vi "Rio_Testing_MoveXY (DONE).vi"() -> ()   [LabVIEW 2017]
panel:
  out "Counter Out 2":i32
  out "Counter Out":i32
  in  "Stop Button":bool
  in  "Boolean":bool
  out "Waveform Chart 2":dbl[][](graph)
  out "Waveform Chart":dbl[][](graph)
  out "Output Charts":T1
  in  "Home Position":dbl[](array[numeric])
  in  "Error In":errorcluster
  in  "Home/Coordinate (T/F)":bool
  in  "Coordinate":dbl[](array[numeric])
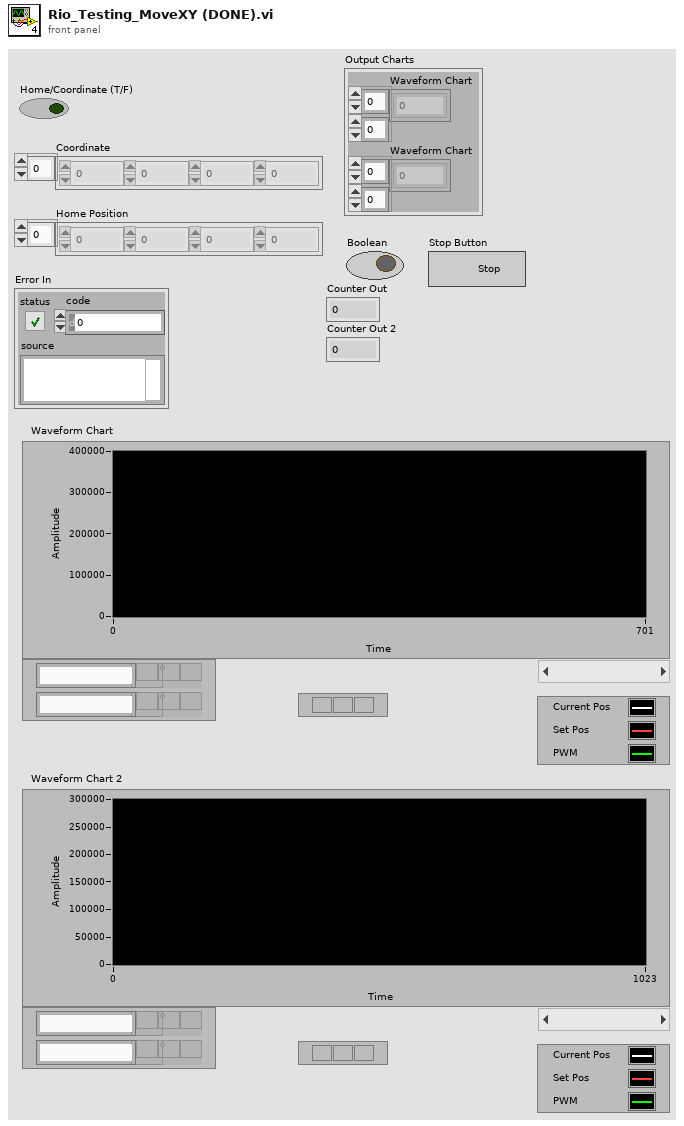
[diagram p1: front panel]
types:
  T1 = cluster{"Waveform Chart":dbl[][], "Waveform Chart":dbl[][]}
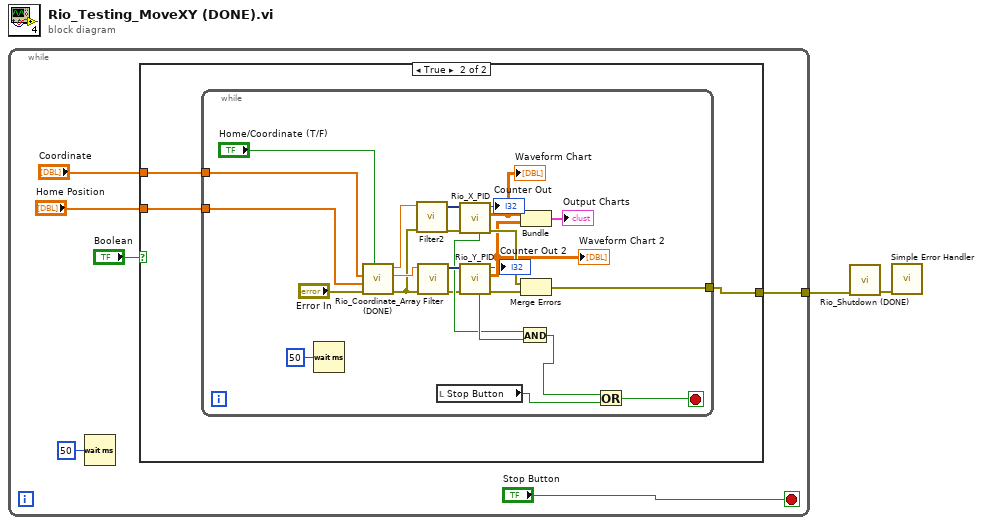
[diagram p0: block diagram]
diagram:
  n1 = while {
    tunnel: [w6] -> w1
    stop <- "Stop Button" stop-if-true
    n2 = Wait (ms)(milliseconds to wait=u32 50) -> ()  [unwired: 1 out]
    n3 = case shown="True" "Boolean" {
      tunnel: [_ w11] -> w6
      tunnel: "Home Position" -> [_ w10]
      tunnel: "Coordinate" -> [_ w9]
      frame False {
      }
      frame True {
        n4 = while {
          tunnel: [w22] -> w11
          tunnel: w10 -> [w19]
          tunnel: w9 -> [w18]
          stop <- w15 stop-if-true
          n5 = Wait (ms)(milliseconds to wait=u32 50) -> ()  [unwired: 1 out]
          n6 = call "Rio_Coordinate_Array (DONE).vi"("Coordinate Selection"="Home/Coordinate (T/F)", "Error In"="Error In", "Home Position"=w19, "Coordinate"=w18) -> ("Error Out"=w24:errorcluster, "Y"=w35:dbl, "X"=w23:dbl)  [unwired: 5 in]
          n7 = call "Filter2"("error in (no error)"=w24, "Signal"=w23) -> ("error out"=w25:errorcluster, "Filtered Signal"=w26:dynamicdata)  [unwired: 8 in]
          n8 = call "Filter"("error in (no error)"=w24, "Signal"=w35) -> ("error out"=w28:errorcluster, "Filtered Signal"=w33:dynamicdata)  [unwired: 8 in]
          n9 = local read "Stop Button"() -> (w14:bool)
          n10 = call "Rio_X_PID.vi"("Error In"=w25, "Setpoint"=w26) -> ("Error Out"=w29:errorcluster, "Waveform Chart"=w21:dbl[][], "Counter Out"=→"Counter Out":i32, "Stop"=w31:bool)  [unwired: 6 in]
          "Waveform Chart" <- w21
          n11 = call "Rio_Y_PID.vi"("Error In"=w28, "Setpoint"=w33) -> ("Error Out"=w30:errorcluster, "Waveform Chart"=w20:dbl[][], "Counter Out"=→"Counter Out 2":i32, "Stop"=w32:bool)  [unwired: 6 in]
          "Waveform Chart 2" <- w20
          n12 = And(x=w31, y=w32) -> (x .and. y?=w16:bool)
          n13 = Bundle("Waveform Chart"=w21, "Waveform Chart"=w20) -> (→"Output Charts":T1)  [unwired: 1 in]
          n14 = Merge Errors(w29, w30) -> (w22:errorcluster)
          n15 = Or(x=w16, y=w14) -> (x .or. y?=w15:bool)
        }
      }
    }
  }
  n16 = call "Rio_Shutdown (DONE).vi"("error in (no error)"=w1) -> ("error out"=w2:errorcluster)  [unwired: 10 in]
  n17 = call <vilib>:"Simple Error Handler.vi"("error in (no error)"=w2) -> ()  [unwired: 4 in, 5 out]
